vi "Packet_decode_Int32.vi"(9 "StartByte":i32, 11 "RawData":u8[](array[numeric])) -> (1 "NextByte":i32, 3 "Int32_Value":i32)   [LabVIEW 2019, in "PhotonVisionLib.lvlib"]
doc: "Decode (or strip out) a 32 bit integer value from the provided byte array. No conversion or decoding is actually done, the memory is just copied, and the value is cast to the correct type.\n\nInputs\n - RawData -- Array of bytes containing the data to be extracted.\n - StartByte -- The starting byte number (the first byte starts at 0)\n\nOutputs\n - INT32_Value -- Extracted 32 bit integer value.\n - NextByte -- The starting byte index for the next value (regardless of type)."
uses:
  PhotonVisionLib.lvlib
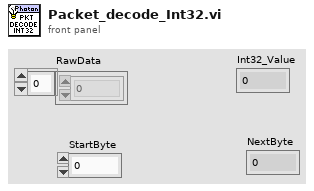
[diagram p1: front panel]
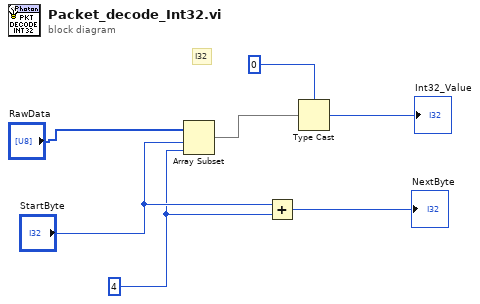
[diagram p0: block diagram]
diagram:
  w1 = 4 ("length")
  # "I32"
  n1 = Array Subset(array="RawData", index="StartByte", length=w1) -> (w5:u8[])
  n2 = Add(x="StartByte", y=w1) -> (x+y=→"NextByte":i32)
  n3 = Type Cast(type=0, x=w5) -> (*(type *) &x=→"Int32_Value":i32)
